vi "Read Ignore Past Updates.vi"(11 "SubscriptionPolicy in":refnum<class "SubscriptionPolicy.lvclass">) -> (2 "Ignore Past Updates?":bool)   [LabVIEW 2015, in "IMediator.lvlib" / "SubscriptionPolicy.lvclass"]
uses:
  SubscriptionPolicy.lvclass
  SubscriptionPolicy.lvclass/SubscriptionPolicy.ctl
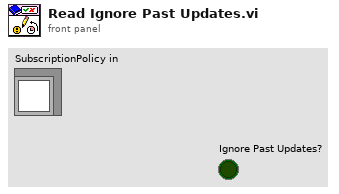
[diagram p1: front panel]
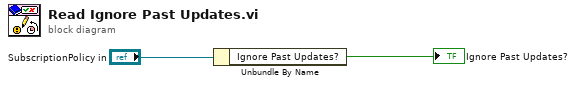
[diagram p0: block diagram]
diagram:
  n1 = Unbundle By Name("SubscriptionPolicy in") -> ("Ignore Past Updates?"=→"Ignore Past Updates?":bool)
